vi "Contains Sub-Index.vi"(8 "Error In":errorcluster, 10 "Sub-Index":u8, 11 "reference in":refnum<class "OD Entry.lvclass">) -> (0 "Error Out":errorcluster, 2 "Contains?":bool, 3 "reference out":refnum<class "OD Entry.lvclass">)   [LabVIEW 2019, in "Electronic Datasheet.lvlib" / "OD Entry.lvclass"]
doc: "Returns true if the object contains a subindex"
uses:
  OD Entry.lvclass
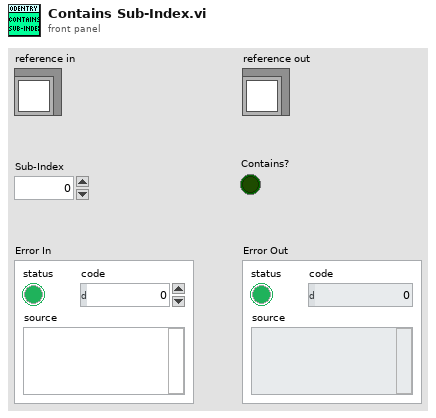
[diagram p1: front panel]
types:
  T1 = typedef "Electronic Datasheet.lvlib/OD Entry.lvclass/ObjectAttributes.ctl" = cluster{"Index":u16, "ObjectType":refnum<class "Object Type Base.lvclass">, "Denotation":string, "Count":u8, "ObjExtend":u8, "Label":string, "Description":string, "PDO Mapping Type":T2, "Sub-Entries":map{u8, refnum<class "OD Sub-Entry.lvclass">}}
  T2 = typedef "Electronic Datasheet.lvlib/PDO Mapping Type.ctl" = enum16{"no", "optional", "RPDO", "TPDO", "UNKNOWN"}
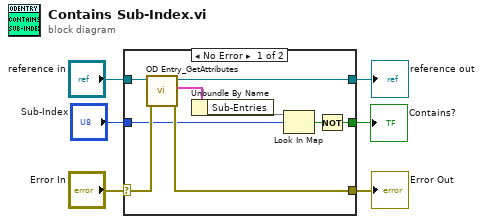
[diagram p0: block diagram]
diagram:
  n1 = case shown="No Error" "Error In" {
    selector: "Error In" -> [w15 w17]
    tunnel: [w14 w17] -> w5
    tunnel: "reference in" -> [w13 w16]
    tunnel: [w12 w16] -> w3
    tunnel: "Sub-Index" -> [w11 _]
    tunnel: [w7 _] -> w1
    frame No Error {
      n2 = call "OD Entry_GetAttributes.vi"("Error In"=w15, "reference in"=w13) -> ("Error Out"=w14:errorcluster, "Data"=w9:T1, "reference out"=w12:refnum<class "OD Entry.lvclass">)  [unwired: 6 in, 1 out]
      n3 = Unbundle By Name(w9) -> ("Sub-Entries"=w8:map{u8, refnum<class "OD Sub-Entry.lvclass">})
      n4 = Look In Map(map=w8, key=w11) -> (key not found?=w10:bool)  [unwired: 1 in, 1 out]
      n5 = Not(x=w10) -> (.not. x?=w7:bool)
    }
    frame Error {
    }
  }
  "Error Out" <- w5
  "reference out" <- w3
  "Contains?" <- w1
